vi "TIO Stream Read Non-blocking_Ser.vi"(8 "error in (no error)":errorcluster, 11 "Nom de ressource VISA":refnum<visa-resource-name>) -> (0 "error out":errorcluster, 1 "Payload":string, 2 "Type":u16(ring)=2 items=["Invalid", "Log", "RPC Request", "RPC Reply", "RPC Error", "Stream Description", "User"], 3 "Nom de ressource VISA Out":refnum<visa-resource-name>, 4 "Data Ok":bool)   [LabVIEW 2012]
uses:
  <userlib>/TIO Library 2010/TIO Serial Checksum CRC32.vi
panel:
  out "Routing Size":u8
  out "Payload Length":u16
  # "TODO Handle routing"
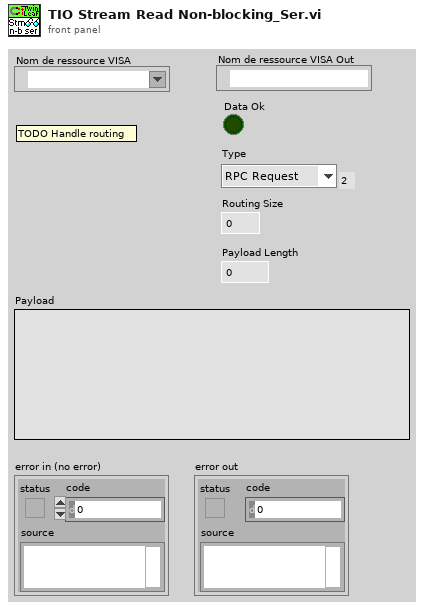
[diagram p1: front panel]
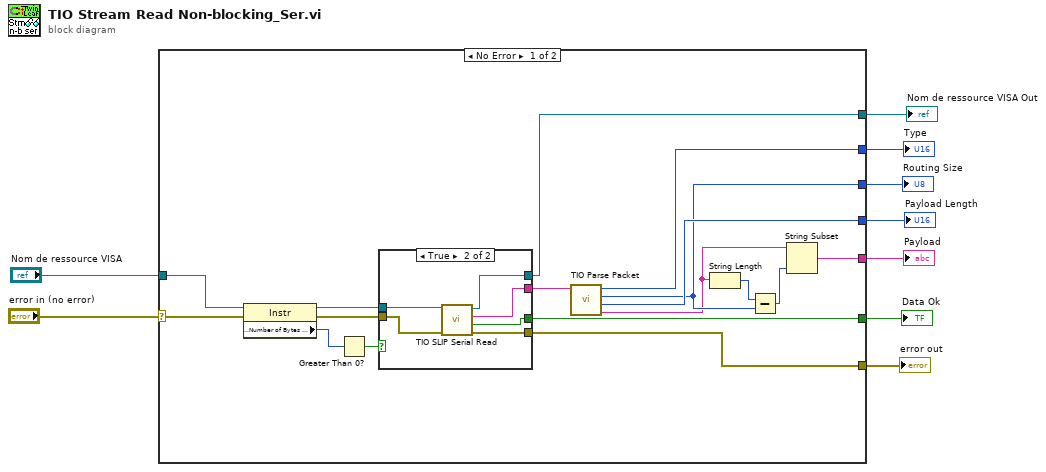
[diagram p0: block diagram]
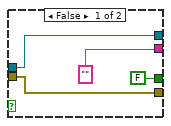
[diagram p2: hidden frame]
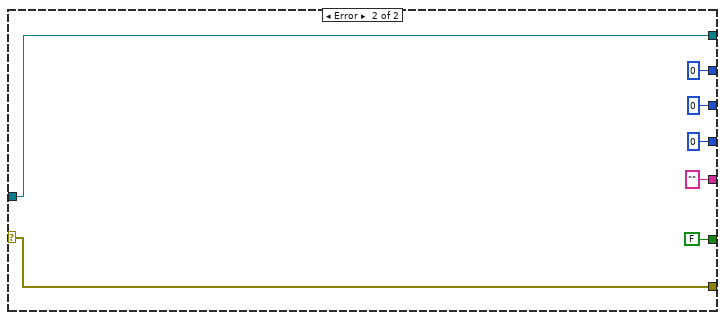
[diagram p3: hidden frame]
diagram:
  n1 = case shown="No Error" "error in (no error)" {
    selector: "error in (no error)" -> [w10 w43]
    tunnel: [w26 w43] -> w9
    tunnel: [w25 u16 0 ("Payload Length")] -> w8
    tunnel: [w24 u16 0 ("Type")] -> w7
    tunnel: [w22 u8 0 ("Routing Size")] -> w6
    tunnel: [w19 "" ("Payload")] -> w5
    tunnel: [w13 FALSE ("CRC32")] -> w4
    tunnel: "Nom de ressource VISA" -> [w12 w42]
    tunnel: [w11 w42] -> w2
    frame No Error {
      n2 = property class="Instr"(reference=w12, error in=w10) -> (reference out=w17:refnum<visa-resource-name>, error out=w16:errorcluster, "Serial Settings:Number of Bytes at Serial Port"=w15:u32)
      n3 = Greater Than 0?(x=w15) -> (x > 0?=w14:bool)
      n4 = case shown="True" w14 {
        tunnel: [w30 w36] -> w26
        tunnel: ["" ("Payload") w33] -> w18
        tunnel: w17 -> [w27 w35]
        tunnel: w16 -> [w30 w34]
        tunnel: [FALSE ("CRC32") w32] -> w13
        tunnel: [w27 w31] -> w11
        frame False {
        }
        frame True {
          n5 = call <userlib>:"TIO SLIP Serial Read.vi"("error in (no error)"=w34, "VISA resource name"=w35) -> ("error out"=w36:errorcluster, "CRC32"=w32:bool, "Payload"=w33:string, "VISA resource name Out"=w31:refnum<visa-resource-name>)  [unwired: 6 in]
        }
      }
      n6 = call <userlib>:"TIO Parse Packet.vi"("Packet"=w18) -> ("Payload"=w21:string, "Payload Length"=w25:u16, "Routing Size"=w22:u8, "Type"=w24:u16)  [unwired: 7 in]
      n7 = String Length(string=w21) -> (length=w23:i32)
      n8 = Subtract(x=w23, y=w22) -> (x-y=w20:i32)
      n9 = String Subset(string=w21, length (rest)=w20) -> (substring=w19:string)  [unwired: 1 in]
    }
    frame Error {
    }
  }
  "error out" <- w9
  "Payload" <- w5
  "Type" <- w7
  "Routing Size" <- w6
  "Payload Length" <- w8
  "Data Ok" <- w4
  "Nom de ressource VISA Out" <- w2
